vi "Launcher.vi"   [LabVIEW 2024]
uses:
  Startup.vi
  Startup.lvlib
panel:
  # "Launcher"
types:
  T1 = enum32{"Invalid", "Standard", "Closed", "Hidden", "Minimized", "Maximized"}
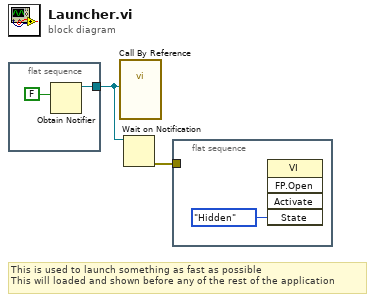
[diagram p0: block diagram]
diagram:
  # "This is used to launch something as fast as possible\nThis will loaded and shown before any of the rest of the application"
  n1 = flat-sequence {
    tunnel: [w3] -> w2
    frame #0 {
      n2 = Obtain Notifier(notification data type=FALSE) -> (notifier out=w3:refnum<notifier>)  [unwired: 3 in, 2 out]
    }
  }
  n3 = call-by-ref "?"("Started"=w2) -> ()  [unwired: 13 in, 2 out]
  n4 = Wait on Notification(notifier=w2) -> (error out=w1:errorcluster)  [unwired: 3 in, 3 out]
  n5 = flat-sequence {
    tunnel: w1 -> [_]
    frame #0 {
      n6 = invoke class="VI" method="FP.Open"("State"=T1."Hidden") -> ()  [unwired: 4 in, 5 out]
    }
  }
